vi "ReadBase.vi"(7 "ConcreteActor":refnum<class "ConcreteActor.lvclass">) -> (3 "Base":T1)   [LabVIEW 2020, in "_Template.lvlib" / "ActorTemplate.lvlib" / "{{Name}}.lvlib" / "ConcreteActor.lvclass"]
uses:
  ConcreteActor.lvclass
  ConcreteActor.lvclass/ConcreteActor.ctl
  jettl/jettl/Actor/Actor.lvclass
  jettl/jettl/Lifecycle.ctl
  jettl/jettl/jettl.lvlib
  jettl/jettl/Message/Message.lvclass
  jettl/jettl/MessageSet.ctl
  jettl/jettl/Messages.ctl
  jettl/jettl/Message.ctl
  jettl/jettl/ActorType.ctl
  jettl/jettl/Actor.ctl
  jettl/jettl/ComponentActorMap.ctl
  jettl/jettl/Base.ctl
  jettl/jettl/TellComponentMap.ctl
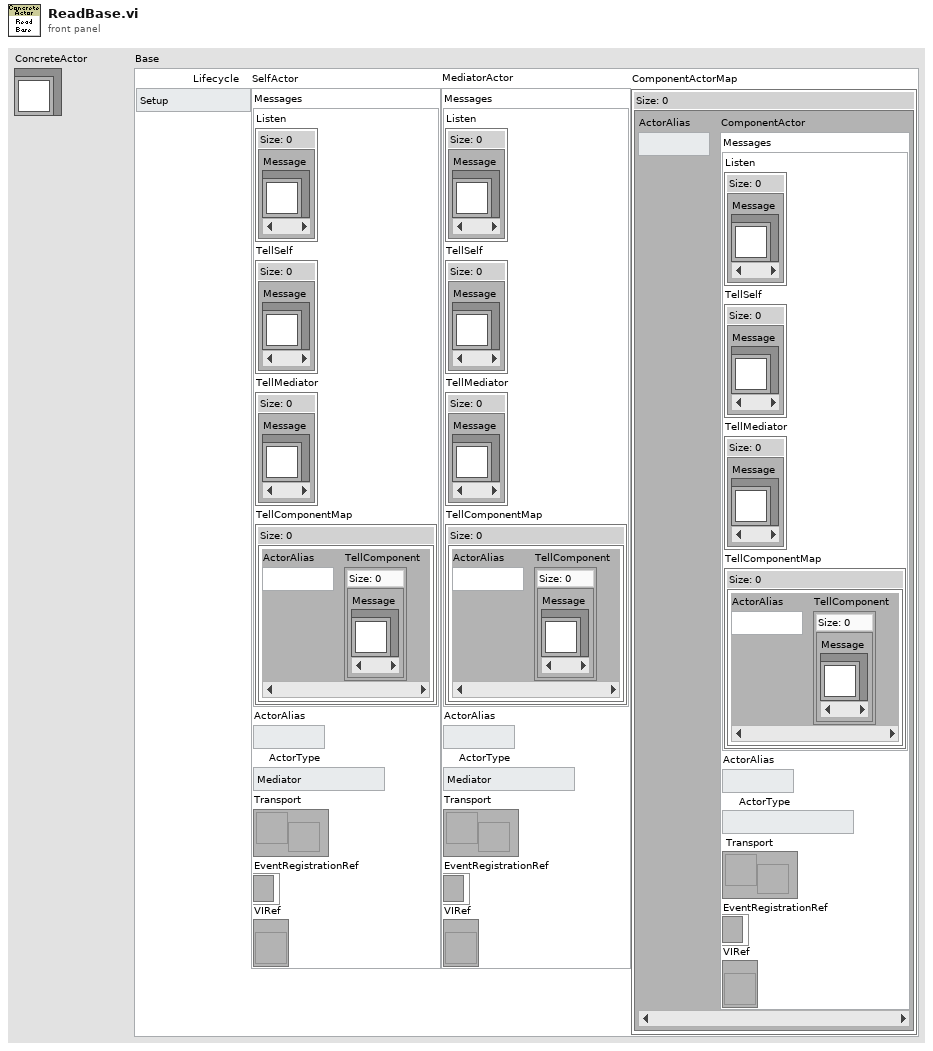
[diagram p1: front panel]
types:
  T1 = typedef "jettl.lvlib/Base.ctl" = cluster{"Lifecycle":T2, "SelfActor":T3, "MediatorActor":T3, "ComponentActorMap":T8}
  T2 = typedef "jettl.lvlib/Lifecycle.ctl" = enum16{"Setup", "TeardownBeforeStart", "Start", "Running", "Stop", "TeardownAfterStart"}
  T3 = typedef "jettl.lvlib/Actor.ctl" = cluster{"Messages":T4, "ActorAlias":string, "ActorType":T7, "Transport":refnum<user-event>, "EventRegistrationRef":refnum<event-registration>, "VIRef":refnum<vi>}
  T4 = typedef "jettl.lvlib/Messages.ctl" = cluster{"Listen":T5, "TellSelf":T5, "TellMediator":T5, "TellComponentMap":T6}
  T5 = typedef "jettl.lvlib/MessageSet.ctl" = set{refnum<class "Message.lvclass">}
  T6 = typedef "jettl.lvlib/TellComponentMap.ctl" = map{string, T5}
  T7 = typedef "jettl.lvlib/ActorType.ctl" = enum16{"Mediator", "Component"}
  T8 = typedef "jettl.lvlib/ComponentActorMap.ctl" = map{string, T3}
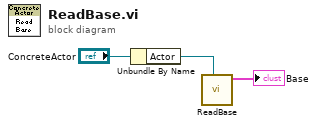
[diagram p0: block diagram]
diagram:
  n1 = Unbundle By Name("ConcreteActor") -> ("Actor"=w2:refnum<class "Actor.lvclass">)
  n2 = call-dynamic "ReadBase.vi"("Actor"=w2) -> ("Base"=→"Base":T1)  [unwired: 10 in]
